vi "CmdConsole.Run and Wait.vi"(8 "error in (no error)":errorcluster, 9 "Timeout(s)":dbl=1.0, 10 "Args":string, 11 "CmdConsole in":refnum<class "CmdConsole.lvclass">) -> (0 "error out":errorcluster, 1 "Std Error":string, 2 "Std Out":string, 3 "CmdConsole out":refnum<class "CmdConsole.lvclass">, 4 "RtnCode":i32, 5 "Duration":dbl)   [LabVIEW 2024, in "CmdConsole.lvclass"]
uses:
  CmdConsole.lvclass
  CmdConsole.lvclass/CmdConsole.ctl
  Errors.lvlib
  <vilib>/KATE/Time/Time Utils.lvlib
panel:
  out "HasExited":bool
  out "WaitForExit":bool
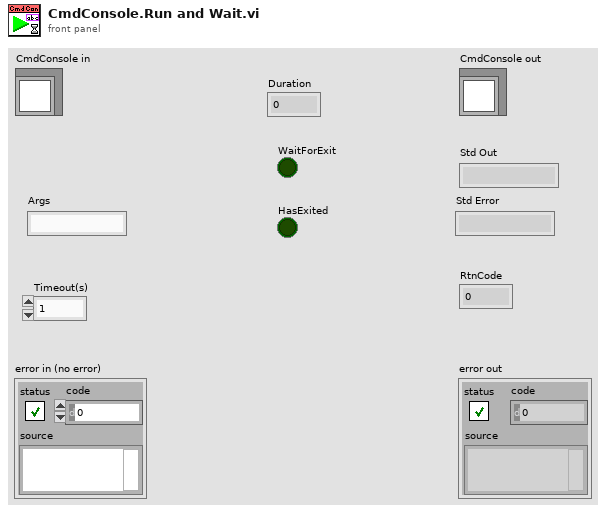
[diagram p1: front panel]
types:
  T1 = cluster{"StdOut":string, "StdErr":string, "RtnCode":i32}
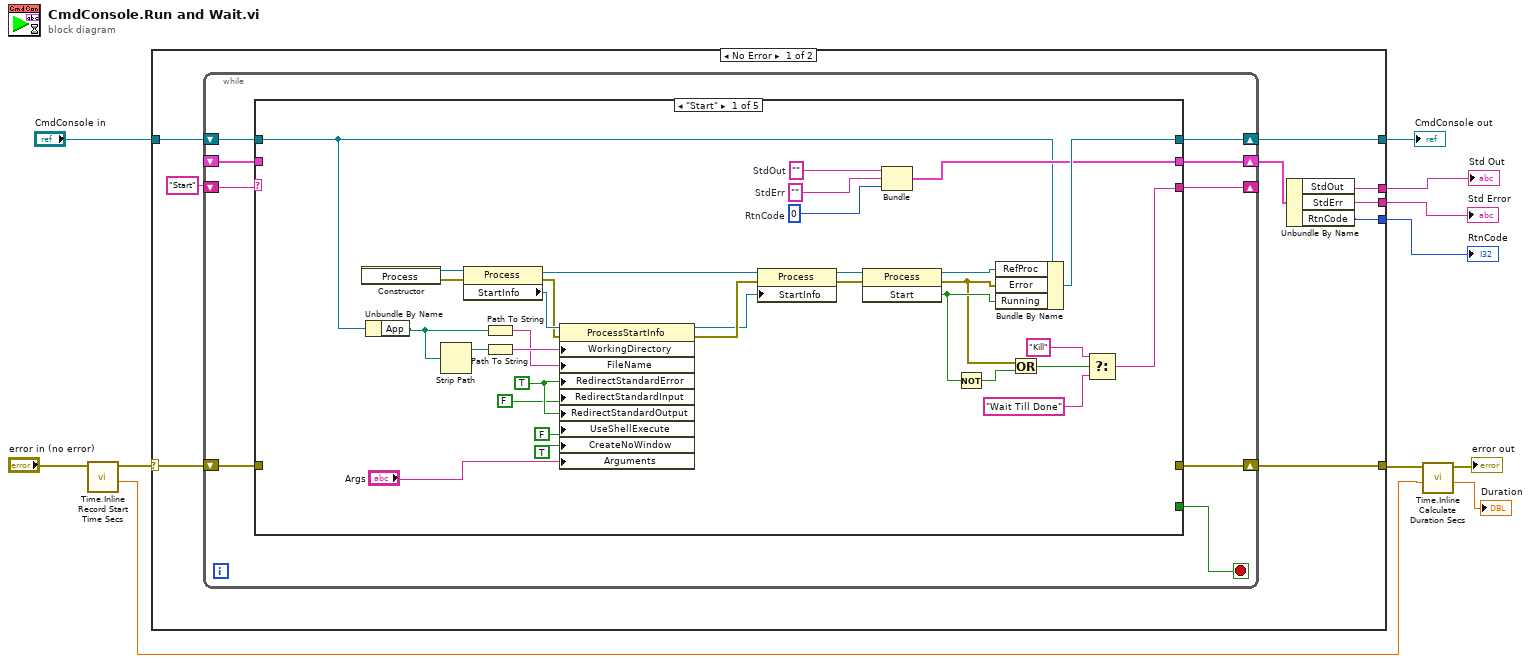
[diagram p0: block diagram]
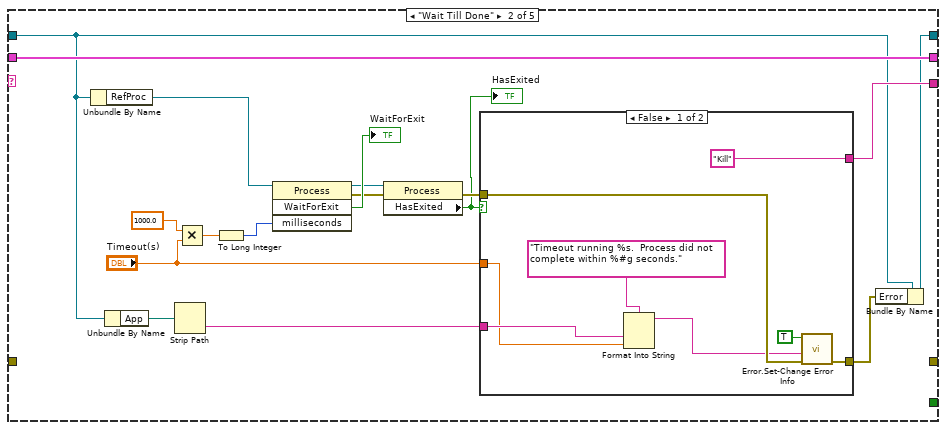
[diagram p2: hidden frame]
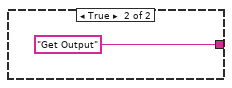
[diagram p3: hidden frame]
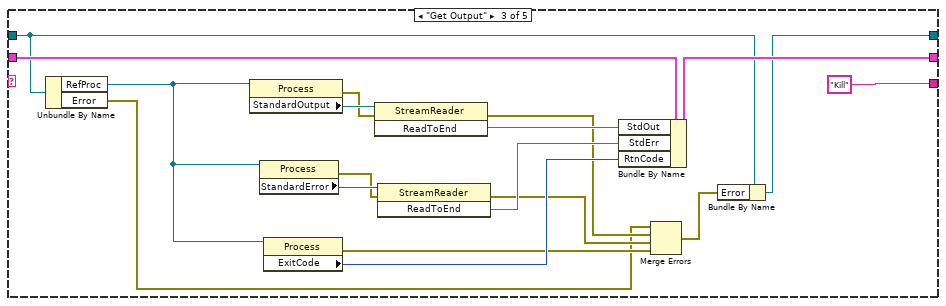
[diagram p4: hidden frame]
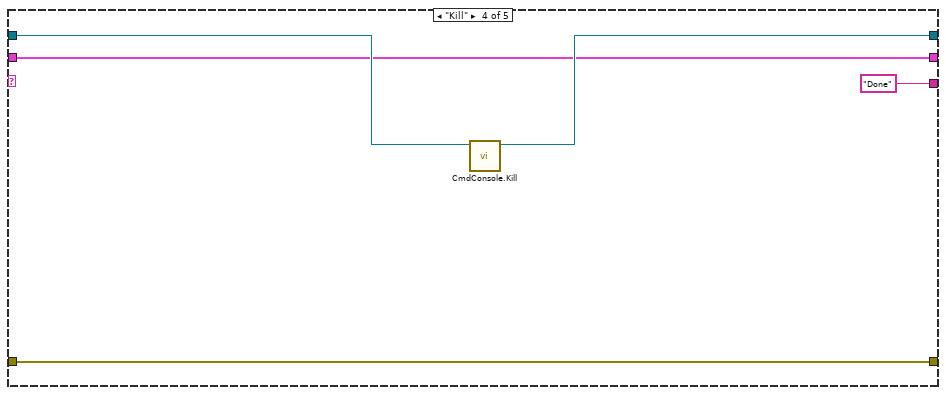
[diagram p5: hidden frame]
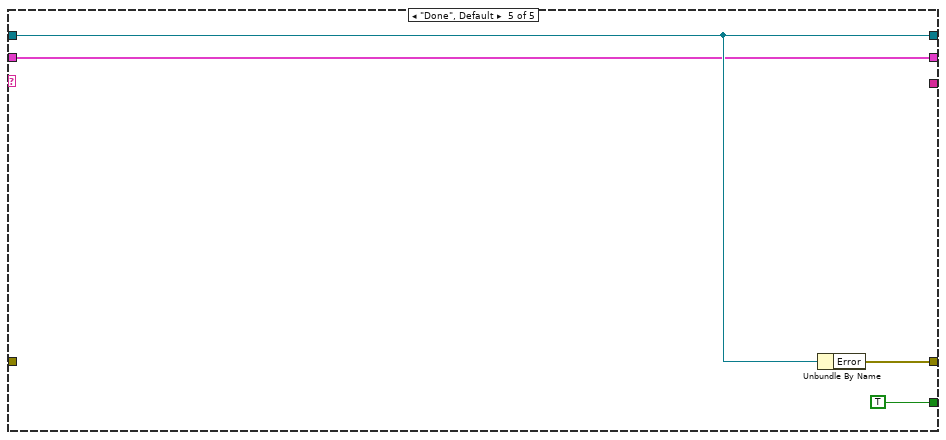
[diagram p6: hidden frame]
diagram:
  n1 = call <vilib>:"Time.Inline Record Start Time Secs.vi"("Error In Upper"="error in (no error)") -> ("Start(s)"=w2:dbl, "Error Out Upper"=w5:errorcluster)  [unwired: 8 in, 1 out]
  n2 = case shown="No Error" w5 {
    selector: w5 -> [w17 w116]
    tunnel: [w18 w116] -> w3
    tunnel: [w16 w115] -> w10
    tunnel: "CmdConsole in" -> [w20 w115]
    tunnel: [w15 _] -> w9
    tunnel: [w13 _] -> w8
    tunnel: [w12 _] -> w7
    frame No Error {
      n3 = while {
        shift-right: [w28] -> w16
        shift-left: w20 -> [w29]
        shift-right: [w26] -> _
        shift-left: "Start" -> [w27]
        shift-right: [w24] -> w18
        shift-left: w17 -> [w21]
        shift-right: [w23] -> w14
        shift-left: _ -> [w22]
        stop <- w25 stop-if-true
        n4 = case shown="\"Start\"" w27 {
          tunnel: w29 -> [w31 w63 w96 w110 w113]
          tunnel: [w45 w62 w95 w108 w113] -> w28
          tunnel: [w37 w74 "Kill" "Done" _] -> w26
          tunnel: [_ _ _ _ TRUE] -> w25
          tunnel: [_ _ _ w106 w112] -> w24
          tunnel: [w32 w69 w101 w107 w111] -> w23
          tunnel: w22 -> [_ w69 w102 w107 w111]
          tunnel: w21 -> [_ _ _ w106 _]
          frame "Start" {
            w33 = 0  # RtnCode
            w34 = ""  # StdErr
            w35 = ""  # StdOut
            w46 = TRUE ("UseShellExecute")
            n5 = constructor class="Process"() -> (reference out=w61:refnum<k24>, error out=w60:errorcluster)  [unwired: 3 in, 1 out]
            n6 = Unbundle By Name(w31) -> ("App"=w47:path)
            n7 = Strip Path(path=w47) -> (stripped path=w50:path)  [unwired: 1 out]
            n8 = property class="Process"(reference=w61, error in=w60) -> (reference out=w53:refnum<k24>, error out=w54:errorcluster, "StartInfo"=w59:refnum<k24>)
            n9 = Path To String(path=w47) -> (string=w48:string)
            n10 = Path To String(path=w50) -> (string=w49:string)
            n11 = property class="ProcessStartInfo"(reference=w59, error in=w54, "WorkingDirectory"=w49, "FileName"=w48, "RedirectStandardError"=w46, "RedirectStandardInput"=FALSE ("UseShellExecute"), "RedirectStandardOutput"=w46, "UseShellExecute"=FALSE, "CreateNoWindow"=TRUE, "Arguments"="Args") -> (reference out=w55:refnum<k24>, error out=w56:errorcluster)
            n12 = property class="Process"(reference=w53, error in=w56, "StartInfo"=w55) -> (reference out=w52:refnum<k24>, error out=w51:errorcluster)
            n13 = invoke class="Process" method="Start"(reference=w52, error in=w51) -> (reference out=w44:refnum<k24>, error out=w41:errorcluster, "Start"=w43:bool)  [unwired: 1 in]
            n14 = Bundle("StdOut"=w35, "StdErr"=w34, "RtnCode"=w33) -> (w32:T1)  [unwired: 1 in]
            n15 = Not(x=w43) -> (.not. x?=w42:bool)
            n16 = Bundle By Name(cluster=w31, "RefProc"=w44, "Error"=w41, "Running"=w43) -> (w45:refnum<class "CmdConsole.lvclass">)
            n17 = Or(x=w41, y=w42) -> (x .or. y?=w40:bool)
            n18 = Select(t="Kill", s=w40, f="Wait Till Done") -> (s? t:f=w37:string)
          }
          frame "Wait Till Done" {
            n19 = Unbundle By Name(w63) -> ("RefProc"=w78:refnum<k24>)
            n20 = Unbundle By Name(w63) -> ("App"=w73:path)
            n21 = Strip Path(path=w73) -> (name=w72:string)  [unwired: 1 out]
            n22 = Multiply(x=1000.0 ("y"), y="Timeout(s)") -> (x*y=w77:dbl)
            n23 = To Long Integer(number=w77) -> (32bit integer=w76:i32)
            n24 = invoke class="Process" method="WaitForExit"(reference=w78, "milliseconds"=w76) -> (reference out=w68:refnum<k24>, error out=w66:errorcluster, "WaitForExit"=→"WaitForExit":bool)  [unwired: 2 in, 1 out]
            n25 = property class="Process"(reference=w68, error in=w66) -> (error out=w67:errorcluster, "HasExited"=w65:bool)  [unwired: 1 out]
            "HasExited" <- w65
            n26 = case shown="False" w65 {
              tunnel: ["Kill" "Get Output"] -> w74
              tunnel: w72 -> [w81 _]
              tunnel: w67 -> [w84 _]
              tunnel: [w83 _] -> w64
              tunnel: "Timeout(s)" -> [w80 _]
              frame False {
                n27 = Format Into String(format string="Timeout running %s.  Process did not complete within %#g seconds.", w81, w80) -> (resulting string=w79:string)  [unwired: 2 in, 1 out]
                n28 = call "Error.Set-Change Error Info.vi"("error in"=w84, "Description"=w79, "Set Error"=TRUE) -> ("error out"=w83:errorcluster)  [unwired: 8 in]
              }
              frame True {
              }
            }
            n29 = Bundle By Name(cluster=w63, "Error"=w64) -> (w62:refnum<class "CmdConsole.lvclass">)
          }
          frame "Get Output" {
            n30 = Unbundle By Name(w96) -> ("RefProc"=w98:refnum<k24>, "Error"=w88:errorcluster)
            n31 = property class="Process"(reference=w98) -> (error out=w94:errorcluster, "StandardOutput"=w104:refnum<k24>)  [unwired: 1 in, 1 out]
            n32 = property class="Process"(reference=w98) -> (error out=w93:errorcluster, "StandardError"=w100:refnum<k24>)  [unwired: 1 in, 1 out]
            n33 = property class="Process"(reference=w98) -> (error out=w92:errorcluster, "ExitCode"=w97:i32)  [unwired: 1 in, 1 out]
            n34 = invoke class="StreamReader" method="ReadToEnd"(reference=w104, error in=w94) -> (error out=w90:errorcluster, "ReadToEnd"=w103:string)  [unwired: 1 in, 1 out]
            n35 = invoke class="StreamReader" method="ReadToEnd"(reference=w100, error in=w93) -> (error out=w91:errorcluster, "ReadToEnd"=w99:string)  [unwired: 1 in, 1 out]
            n36 = Bundle By Name(cluster=w102, "StdOut"=w103, "StdErr"=w99, "RtnCode"=w97) -> (w101:T1)
            n37 = Merge Errors(w88, w90, w91, w92) -> (w89:errorcluster)
            n38 = Bundle By Name(cluster=w96, "Error"=w89) -> (w95:refnum<class "CmdConsole.lvclass">)
          }
          frame "Kill" {
            n39 = call "CmdConsole.Kill.vi"("CmdConsole in"=w110) -> ("CmdConsole out"=w108:refnum<class "CmdConsole.lvclass">)  [unwired: 9 in, 1 out]
          }
          frame "Done", Default {
            n40 = Unbundle By Name(w113) -> ("Error"=w112:errorcluster)
          }
        }
      }
      n41 = Unbundle By Name(w14) -> ("StdOut"=w15:string, "StdErr"=w13:string, "RtnCode"=w12:i32)
    }
    frame Error {
    }
  }
  "CmdConsole out" <- w10
  "Std Error" <- w8
  "RtnCode" <- w7
  "Std Out" <- w9
  n42 = call <vilib>:"Time.Inline Calculate Duration Secs.vi"("Start(Sec)"=w2, "Error In Top"=w3) -> ("Duration(s)"=→"Duration":dbl, "Error Out Top"=→"error out":errorcluster)  [unwired: 7 in, 1 out]
